vi "Agilent Overnight Test.vi"() -> ()   [LabVIEW 2013]
panel:
  in  "sTOP":bool
  in  "file path (use dialog)":path=path "c:/test"
  in  "milliseconds to wait":u32
  out "Waveform Chart":dbl[](graph)
  out "error out 2":errorcluster
  in  "error out":errorcluster
  in  "Com Agilent":refnum<visa-resource-name>
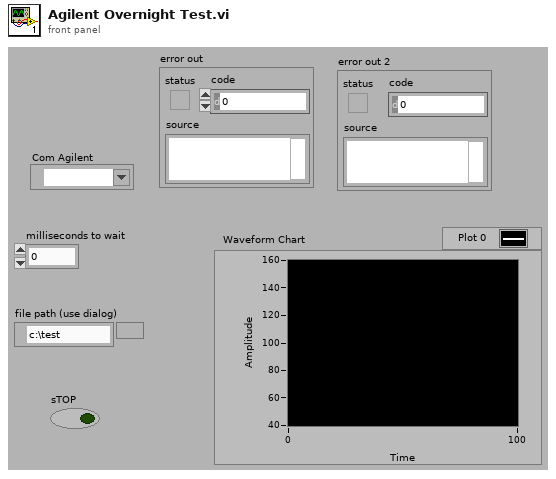
[diagram p1: front panel]
types:
  T1 = enum16{"open", "replace", "create", "open or create", "replace or create", "replace or create with confirmation"}
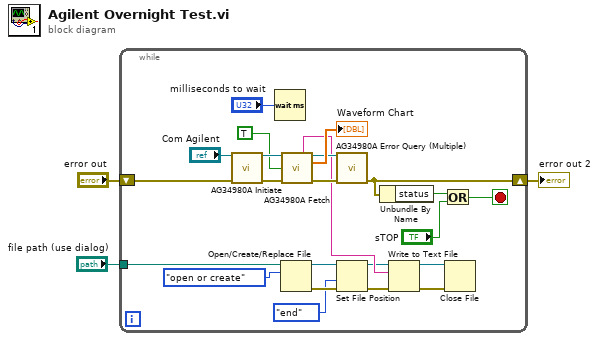
[diagram p0: block diagram]
diagram:
  n1 = while {
    shift-right: [w13] -> w2
    shift-left: "error out" -> [w25]
    tunnel: "file path (use dialog)" -> [w14]
    stop <- w11 stop-if-true
    n2 = call "AG34980A Initiate.vi"("VISA resource name"="Com Agilent", "error in (no error)"=w25) -> ("VISA resource name out"=w21:refnum<visa-resource-name>, "error out"=w23:errorcluster)  [unwired: 12 in]
    n3 = Wait (ms)(milliseconds to wait="milliseconds to wait") -> ()  [unwired: 1 out]
    n4 = Open/Create/Replace File(file path (use dialog)=w14, operation (0:open)=T1."open or create") -> (refnum out=w8:refnum<file>, error out=w5:errorcluster)  [unwired: 4 in, 1 out]
    n5 = call "AG34980A Fetch.vi"("VISA resource name"=w21, "Numbers Only (T:On)"=TRUE, "error in (no error)"=w23) -> ("read buffer"=w17:string, "VISA resource name out"=w20:refnum<visa-resource-name>, "Output Data (Numbers Only)"=→"Waveform Chart":dbl[], "error out"=w22:errorcluster)  [unwired: 8 in, 1 out]
    n6 = call "AG34980A Error Query (Multiple).vi"("VISA resource name"=w20, "error in (no error)"=w22) -> ("error out"=w13:errorcluster)  [unwired: 10 in, 3 out]
    n7 = Set File Position(refnum=w8, from (0:start)=enum16{"start", "end", "current"}."end", error in=w5) -> (refnum out=w7:refnum<file>, error out=w6:errorcluster)  [unwired: 1 in]
    n8 = Unbundle By Name(w13) -> ("status"=w12:bool)
    n9 = Write to Text File(file (use dialog)=w7, text=w17, error in=w6) -> (refnum out=w15:refnum<file>, error out=w16:errorcluster)  [unwired: 1 in, 1 out]
    n10 = Or(x=w12, y="sTOP") -> (x .or. y?=w11:bool)
    n11 = Close File(refnum=w15, error in=w16) -> ()  [unwired: 2 out]
  }
  "error out 2" <- w2
